vi "Data Publishing Service.vi"(10 "NIVS.Workspace Event":refnum<event-registration>, 11 "NIVS.Gateway IP Address":string="localhost") -> ()   [LabVIEW 2019, in "Data Publishing Service.lvlib"]
uses:
  Data Publishing Service.lvlib
  Types/State Variables.ctl
  Types/INI Configuration.ctl
  <vilib>/NI VeriStand/Execution/Workspace/WorkspaceAPI.ctl
  <vilib>/NI VeriStand/Execution/AlarmManager/AlarmManagerAPI.ctl
  <vilib>/Skyline/Tag/Wrapper/Wrapper_class/NI Skyline Tag.lvclass
  <vilib>/NI VeriStand/Execution/Alarm/AlarmAPI.ctl
  <vilib>/Platform/TimedLoop/XDataNode/timing_clust.ctl
  <vilib>/Platform/TimedLoop/XDataNode/nitl_modes.ctl
  <vilib>/Platform/TimedLoop/XDataNode/wakeup.ctl
  <vilib>/Skyline/Tag/Shared/typedefs/DataType.ctl
  <vilib>/Utility/error.llb/DialogType.ctl
  <vilib>/Skyline/Tag/Wrapper/Wrapper_class/Delete Tag (Multiple).vi
  <vilib>/platform/TimedLoop/XDataNode/XDataNode.xnode
  <vilib>/NI VeriStand/Execution/Workspace/NI_VS Workspace ExecutionAPI.lvlib
  <vilib>/Platform/TimedLoop/XDataNode/XDNodeRunTimeDep.lvlib
  <vilib>/Utility/SystemLogging/NI_SystemLogging.lvlib
  NationalInstruments.VeriStand.ClientAPI
  <vilib>/NI VeriStand/Execution/AlarmManager/NI_VS AlarmManager ExecutionAPI.lvlib
  <vilib>/NI VeriStand/Execution/Alarm/NI_VS Alarm ExecutionAPI.lvlib
  <vilib>/Skyline/Tag/Shared/NI Skyline Tag.lvlib
panel:
  out "Loop Rate":u32
  in  "Stop":bool
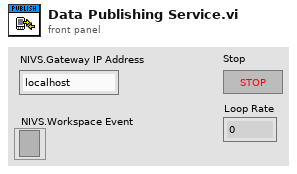
[diagram p1: front panel]
types:
  T1 = typedef "Data Publishing Service.lvlib/State Variables.ctl" = cluster{"INI":T2, "VS.Workspace.Ref":T3, "VS.AlarmManager.Ref":T4, "VS.Connected?":bool, "Tags.Deployed?":bool, "Tags.Initialized":bool, "Process.Name":string, "Aliases":string[], "Alias.Names":string[], "Alias.Tag.Paths":string[], "Alias.SysLink.Refs":refnum<class "NI Skyline Tag.lvclass">[], "Alarms":string[], "Alarm.Names":string[], "Alarm.Tag.Paths":string[], "Alarm.SysLink.Refs":refnum<class "NI Skyline Tag.lvclass">[], "Alarm.VS.Refs":T5[]}
  T2 = typedef "Data Publishing Service.lvlib/INI Configuration.ctl" = cluster{"Library.Name":string, "Alias.FolderPath":string, "Publish.Period_ms":u32, "Alias.Publish":bool, "Alarm.Publish":bool}
  T3 = typedef "NI_VS Workspace ExecutionAPI.lvlib/WorkspaceAPI.ctl" = refnum<k24>
  T4 = typedef "NI_VS AlarmManager ExecutionAPI.lvlib/AlarmManagerAPI.ctl" = refnum<k24>
  T5 = typedef "NI_VS Alarm ExecutionAPI.lvlib/AlarmAPI.ctl" = refnum<k24>
  T6 = typedef "NI_VS Workspace ExecutionAPI.lvlib/SystemStateEventRef.ctl" = cluster{"CustDatRef":refnum<user-event>, "EvtRef":refnum<k27>, "Target State User Event":refnum<user-event>}
  T7 = typedef "NI_VS Workspace ExecutionAPI.lvlib/SystemStateRegEventRef.ctl" = refnum<event-registration>
  T8 = cluster{"NIVS.Workspace Event":refnum<event-registration>, "SystemChangeEventRef":T7}
  T9 = typedef "XDNodeRunTimeDep.lvlib/timing_clust.ctl" = cluster{"Expected End [f-1]":u64, "Actual End [f-1]":u64, "Finished Late? [f-1]":bool, "Expected End [i-1]":u64, "Actual End [i-1]":u64, "Finished Late? [i-1]":bool, "Expected Start [i]":u64, "Actual Start [i]":u64, "Expected Start [f]":u64, "Actual Start [f]":u64, "Source Name":string, "Structure Name":string, "Period":i64, "Deadline":i64, "Offset":i64, "Start":i64, "Priority":i32, "Timeout":i32, "Mode":T10, "Wakeup Reason":T11, "Error":errorcluster, "Source Type":string, "Secondary Source Type":string, "Global End Time":u64, "Global Start Time":u64, "Frame Duration":u64, "Iteration Duration":u64, "Assigned CPU":i32, "I/O Scan Engine Mode":u32}
  T10 = typedef "XDNodeRunTimeDep.lvlib/nitl_modes.ctl" = enum32{"No Change", "Process missed periods, maintain original phase", "Discard missed periods, maintain original phase", "Process missed periods, ignore original phase", "Discard missed periods, ignore original phase"}
  T11 = typedef "XDNodeRunTimeDep.lvlib/wakeup.ctl" = enum32{"Normal", "Aborted", "Asynchronous wakeup", "Timing source error", "Timed loop error", "Timeout"}
  T12 = typedef "NI Skyline Tag.lvlib/DataType.ctl" = enum32{"Double", "I32", "String", "Boolean", "U64", "Timestamp"}
  T13 = typedef "NI_VS Workspace ExecutionAPI.lvlib/SystemState.ctl" = u8
  T14 = typedef "DialogType.ctl" = u16
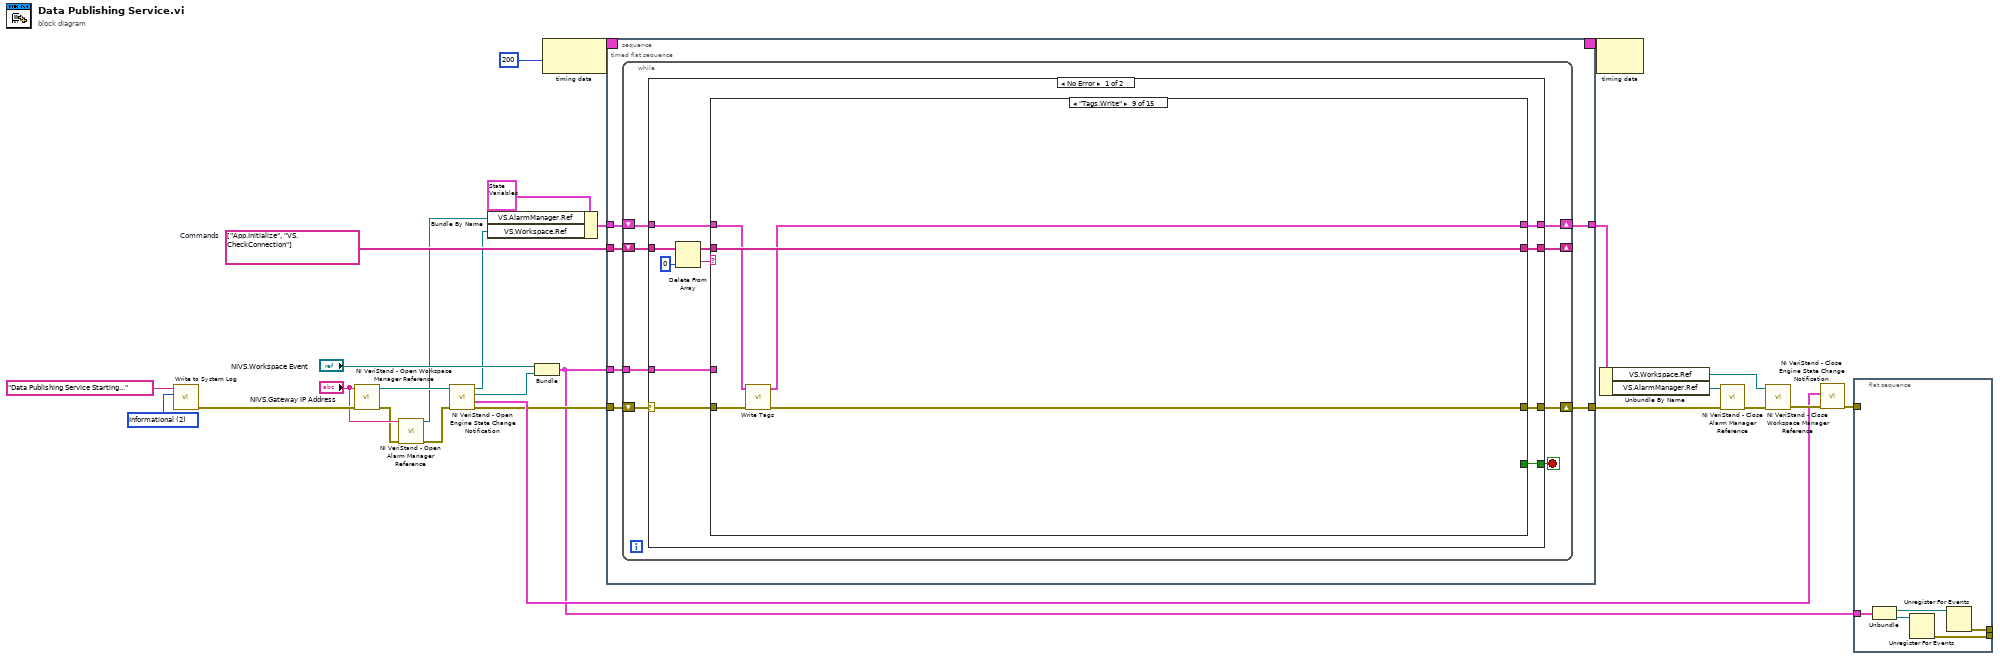
[diagram p0: block diagram]
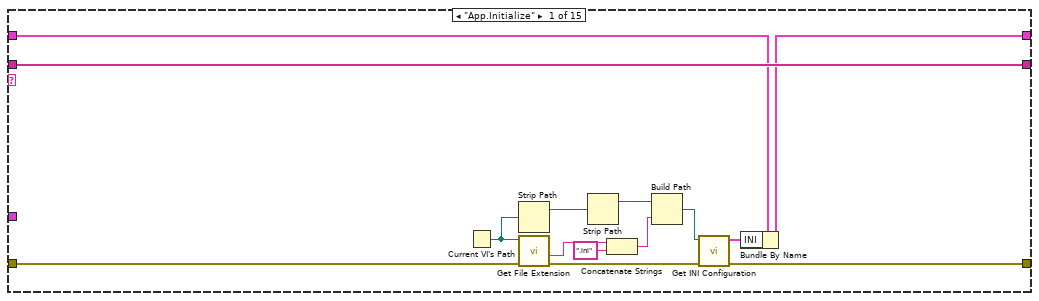
[diagram p2: hidden frame]
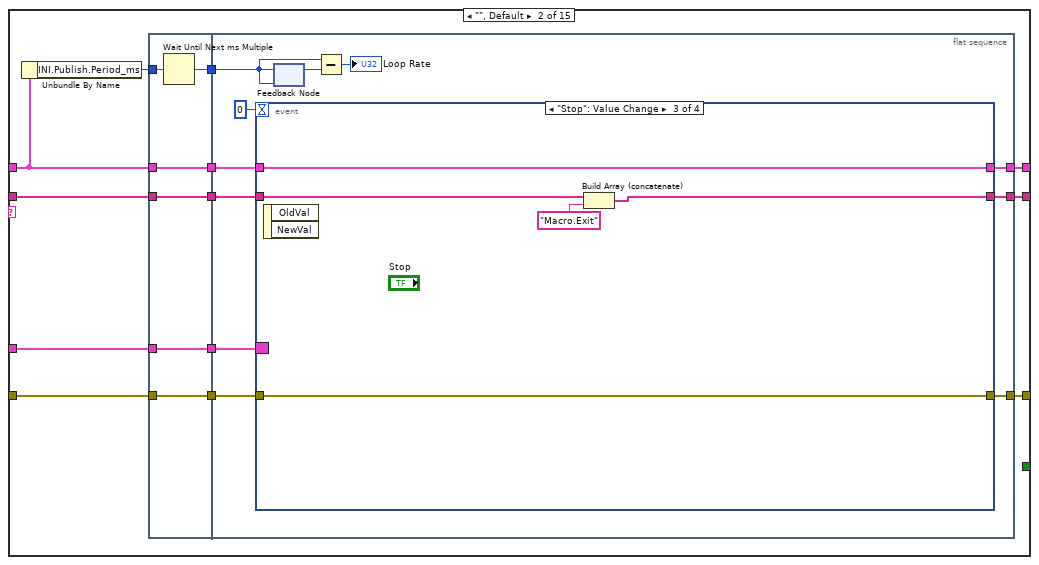
[diagram p3: hidden frame]
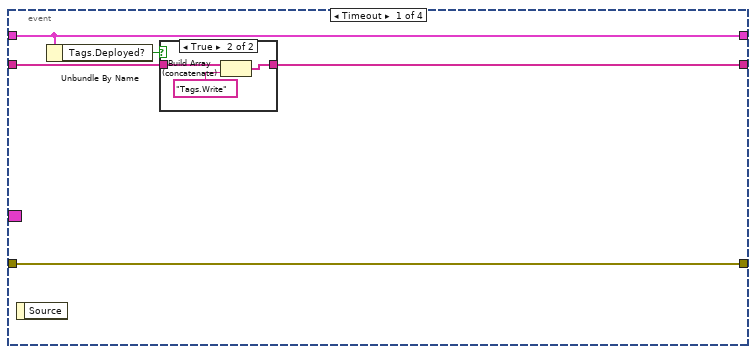
[diagram p4: hidden frame]
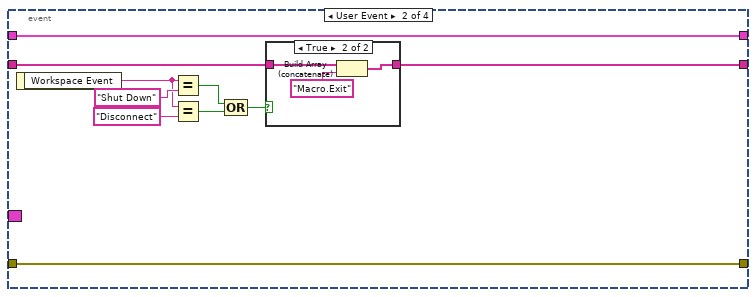
[diagram p6: hidden frame]
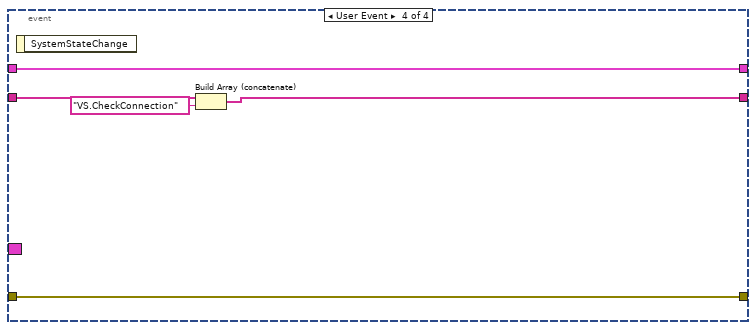
[diagram p8: hidden frame]
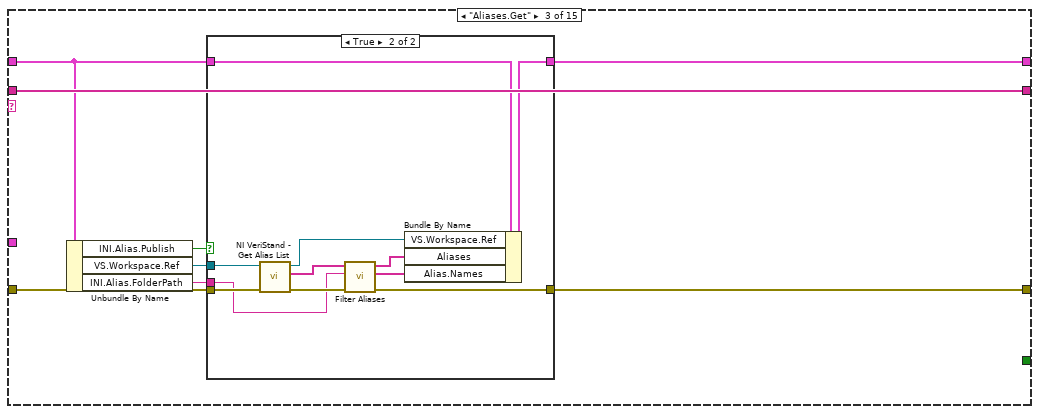
[diagram p9: hidden frame]
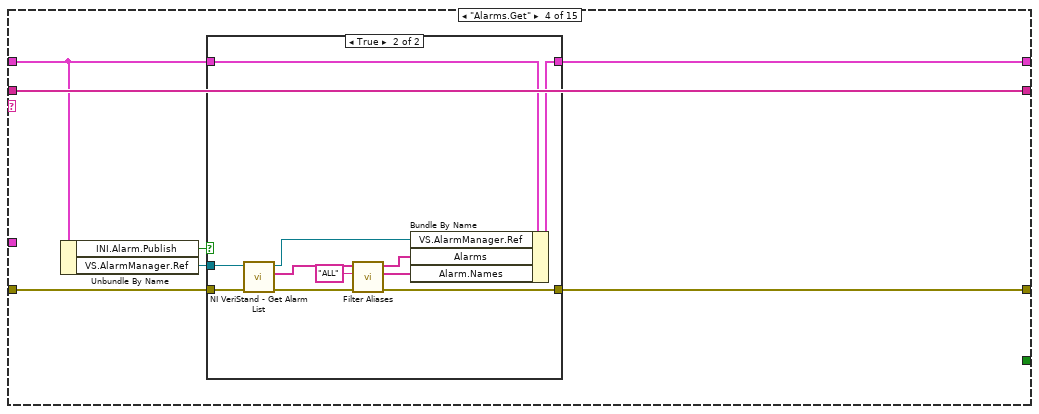
[diagram p11: hidden frame]
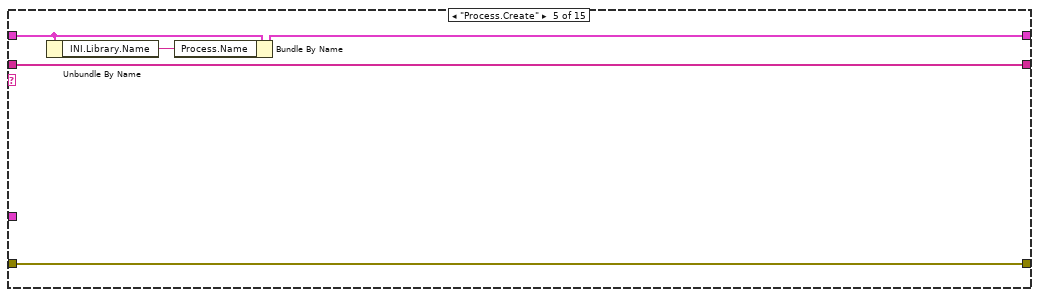
[diagram p13: hidden frame]
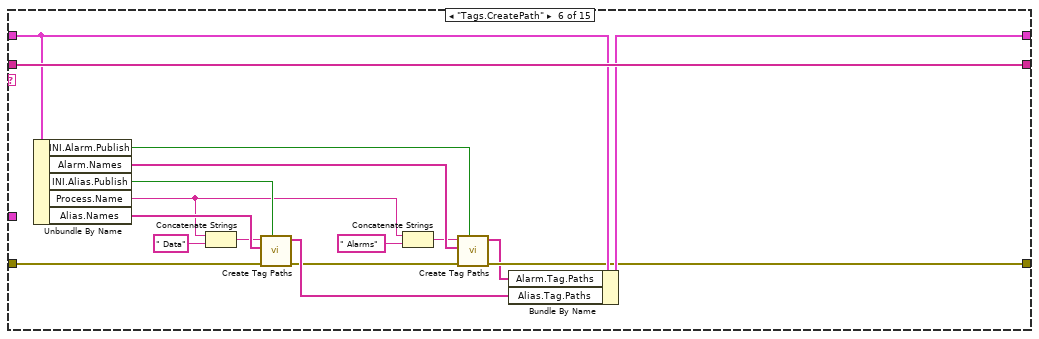
[diagram p14: hidden frame]
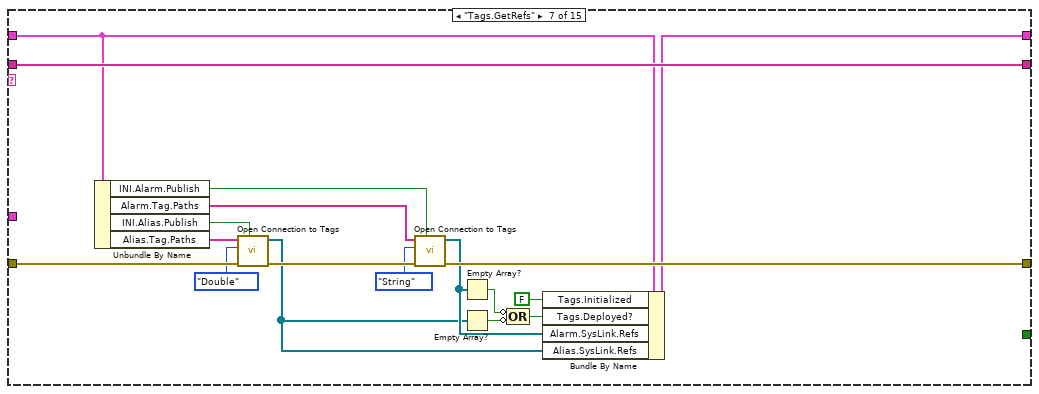
[diagram p15: hidden frame]
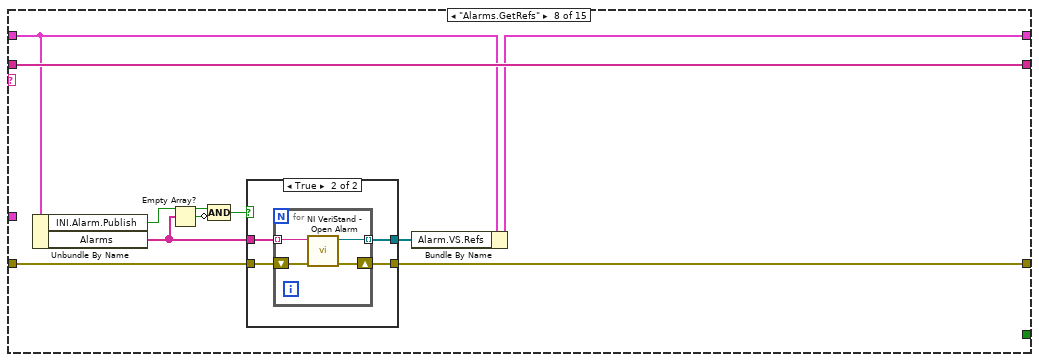
[diagram p16: hidden frame]
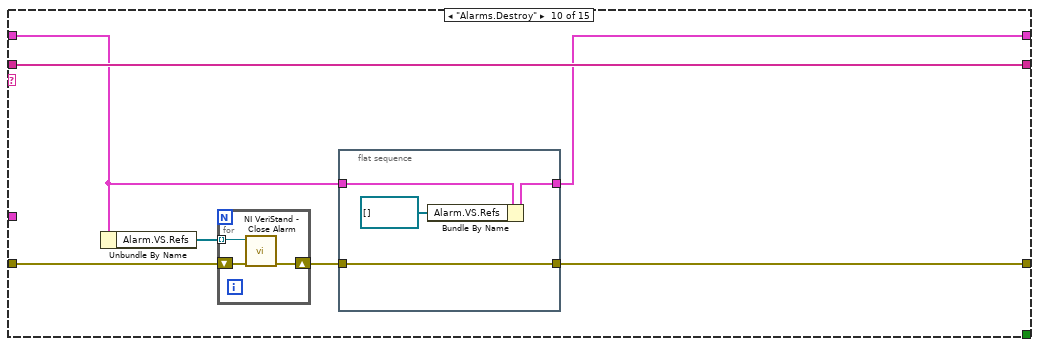
[diagram p18: hidden frame]
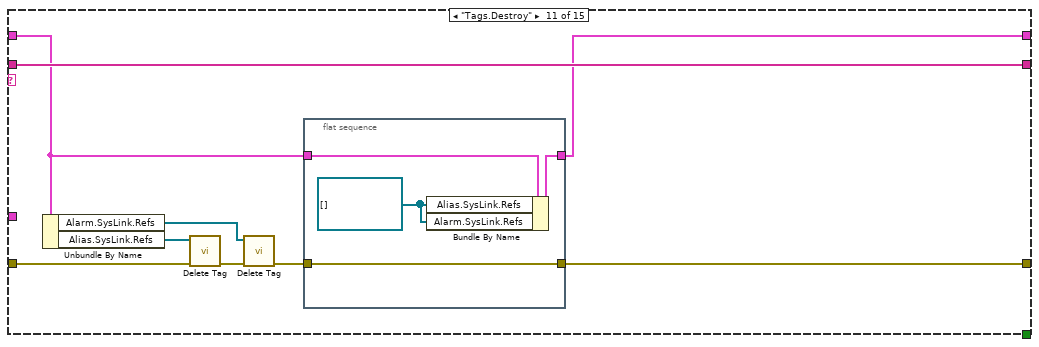
[diagram p19: hidden frame]
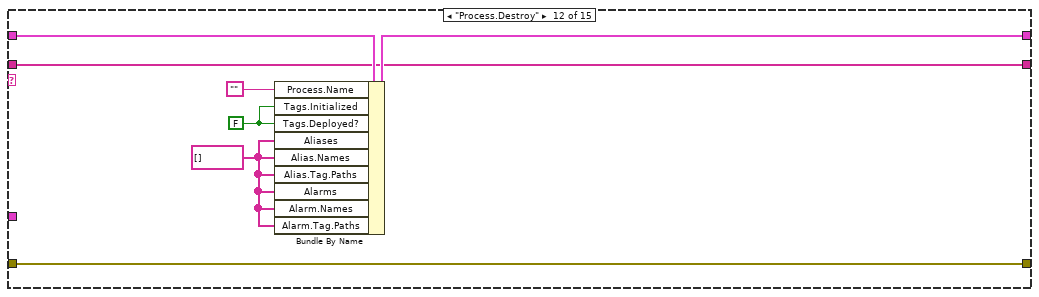
[diagram p20: hidden frame]
diagram:
  w9 = 2 items=["Error", "Warning", "Informational"] ("severity")
  w21 = string[] ["App.Initialize", "VS.CheckConnection"]  # Commands
  n1 = call <vilib>:"Write to System Log.vi"("severity"=w9, "message"="Data Publishing Service Starting...") -> ("error out"=w8:errorcluster)  [unwired: 9 in]
  n2 = call <vilib>:"NI VeriStand - Open Workspace Manager Reference.vi"("error in (no error)"=w8, "Gateway IP Address (\"\": localhost)"="NIVS.Gateway IP Address") -> ("error out"=w6:errorcluster, "WorkspaceManager"=w27:T3)  [unwired: 8 in]
  n3 = call <vilib>:"NI VeriStand - Open Alarm Manager Reference.vi"("error in (no error)"=w6, "Gateway IP Address (\"\": localhost)"="NIVS.Gateway IP Address") -> ("error out"=w5:errorcluster, "AlarmManager"=w4:T4)  [unwired: 8 in]
  n4 = call <vilib>:"NI VeriStand - Open Engine State Change Notification.vi"("error in (no error)"=w5, "WorkspaceManager in"=w27) -> ("error out"=w22:errorcluster, "SystemStateRefs"=w25:T6, "SystemChangeEventRef"=w23:T7, "WorkspaceManager out"=w18:T3)  [unwired: 6 in]
  n5 = Bundle By Name(cluster=T1 {"INI"={"Library.Name"="NI VeriStand Published Data", "Alias.FolderPath"="All", "Publish.Period_ms"=0, "Alias.Publish"=FALSE, "Alarm.Publish"=FALSE}, "VS.Workspace.Ref"=refnum, "VS.AlarmManager.Ref"=refnum, "VS.Connected?"=FALSE, "Tags.Deployed?"=FALSE, "Tags.Initialized"=FALSE, "Process.Name"="", "Aliases"=[], "Alias.Names"=[], "Alias.Tag.Paths"=[], "Alias.SysLink.Refs"=[], "Alarms"=[], "Alarm.Names"=[], "Alarm.Tag.Paths"=[], "Alarm.SysLink.Refs"=[], "Alarm.VS.Refs"=[]}, "VS.AlarmManager.Ref"=w4, "VS.Workspace.Ref"=w18) -> (w16:T1)
  n6 = Bundle("NIVS.Workspace Event"="NIVS.Workspace Event", "SystemChangeEventRef"=w23) -> (w20:T8)  [unwired: 1 in]
  n7 = node-c288(200 ("Priority")) -> (w13:T9)
  n8 = timed-sequence {
    timing: w13 -> [_]
    timing-out: [_] -> w12
    tunnel: [w33] -> w3
    tunnel: w22 -> [w32]
    tunnel: w21 -> [w31]
    tunnel: w20 -> [w30]
    tunnel: w16 -> [w29]
    tunnel: [w28] -> w15
    n9 = timed-flat-sequence {
      tunnel: [w39] -> w33
      tunnel: w32 -> [w38]
      tunnel: w31 -> [w37]
      tunnel: w30 -> [w36]
      tunnel: w29 -> [w35]
      tunnel: [w34] -> w28
      n10 = while {
        tunnel: w36 -> [w47]
        shift-right: [w46] -> w39
        shift-left: w38 -> [w44]
        shift-right: [w41] -> w34
        shift-left: w35 -> [w45]
        shift-right: [w42] -> _
        shift-left: w37 -> [w43]
        stop <- w40 stop-if-true
        n11 = case shown="No Error" w44 {
          selector: w44 -> [w54 w316]
          tunnel: w47 -> [w58 _]
          tunnel: [w57 w319] -> w46
          tunnel: [w56 _] -> w40
          tunnel: w45 -> [w55 w325]
          tunnel: w43 -> [w53 w324]
          tunnel: [w49 w324] -> w42
          tunnel: [w48 w325] -> w41
          frame No Error {
            n12 = Delete From Array(array=w53, index=0) -> (deleted portion=w51:string, array with subset deleted=w50:string[])  [unwired: 1 in]
            n13 = case shown="\"Tags.Write\"" w51 {
              tunnel: w58 -> [_ w85 _ _ _ _ _ _ _ _ _ _ _ _ _]
              tunnel: w54 -> [w59 w84 w141 w161 w181 w197 w215 w225 w239 w245 w262 w271 w289 w300 w309]
              tunnel: [w72 w83 w138 w158 w181 w191 w208 w224 w236 w242 w261 w271 w278 w300 w310] -> w57
              tunnel: [_ _ _ _ _ _ _ _ _ _ _ _ _ _ TRUE] -> w56
              tunnel: w55 -> [w70 w79 w140 w160 w178 w196 w207 w223 w237 w244 w259 w274 w287 w303 w313]
              tunnel: w50 -> [w71 w82 w142 w162 w179 w198 w216 w226 w240 w247 w263 w272 w282 w305 w312]
              tunnel: [w71 w81 w142 w162 w179 w198 w216 w226 w240 w247 w263 w272 w283 w304 w312] -> w49
              tunnel: [w68 w80 w143 w163 w180 w194 w206 w221 w238 w243 w258 w273 w286 w303 w313] -> w48
              frame "App.Initialize" {
                n14 = Current VI's Path() -> (path=w63:path)
                n15 = Strip Path(path=w63) -> (stripped path=w62:path)  [unwired: 1 out]
                n16 = call <vilib>:"Get File Extension.vi"("error in (no error)"=w59, "file"=w63) -> ("error out"=w67:errorcluster, "filename without extension"=w66:string)  [unwired: 5 in, 3 out]
                n17 = Strip Path(path=w62) -> (stripped path=w61:path)  [unwired: 1 out]
                n18 = Concatenate Strings(w66, ".ini" ("string")) -> (w64:string)
                n19 = Build Path(base path=w61, name or relative path=w64) -> (appended path=w60:path)
                n20 = call "Get INI Configuration.vi"("error in (no error)"=w67, "configuration file path"=w60) -> ("error out"=w72:errorcluster, "INI"=w69:T2)  [unwired: 8 in]
                n21 = Bundle By Name(cluster=w70, "INI"=w69) -> (w68:T1)
              }
              frame "", Default {
                n22 = Unbundle By Name(w79) -> ("INI.Publish.Period_ms"=w78:u32)
                n23 = flat-sequence {
                  tunnel: w78 -> [w87]
                  tunnel: w79 -> [w88]
                  tunnel: w82 -> [w89]
                  tunnel: w84 -> [w90]
                  tunnel: w85 -> [w91]
                  tunnel: [w91] -> w77
                  tunnel: [w90] -> w76
                  tunnel: [w89] -> w75
                  tunnel: [w88] -> w74
                  tunnel: [w86] -> w73
                  tunnel: [w100] -> w83
                  tunnel: [w98] -> w81
                  tunnel: [w97] -> w80
                  tunnel: w77 -> [w102]
                  tunnel: w76 -> [w101]
                  tunnel: w75 -> [w99]
                  tunnel: w74 -> [w96]
                  tunnel: w73 -> [w93]
                  frame #0 {
                    n24 = Wait Until Next ms Multiple(millisecond multiple=w87) -> (millisecond timer value=w86:u32)
                  }
                  frame #1 {
                    n25 = event shown="[2] \"Stop\": Value Change" {
                      selector: w102 -> [_ _ _ _]
                      dyn-events: _ -> [_ _ _ _]
                      timeout: 0 -> [_ _ _ _]
                      tunnel: w101 -> [w103 w121 w130 w135]
                      tunnel: [w103 w121 w130 w135] -> w100
                      tunnel: w96 -> [w104 w120 w129 w131]
                      tunnel: w99 -> [w105 w119 w128 w134]
                      tunnel: [w106 w117 w127 w133] -> w98
                      tunnel: [w104 w120 w129 w131] -> w97
                      event Timeout {
                        n26 = event-data() -> ()  [unwired: 1 in, 1 out]
                        n27 = Unbundle By Name(w104) -> ("Tags.Deployed?"=w107:bool)
                        n28 = case shown="True" w107 {
                          tunnel: w105 -> [w108 w110]
                          tunnel: [w108 w109] -> w106
                          frame False {
                          }
                          frame True {
                            n29 = Build Array (concatenate)(w110, "Tags.Write" ("y")) -> (w109:string[])
                          }
                        }
                      }
                      event User Event {
                        n30 = event-data() -> ("Workspace Event"=w112:string)  [unwired: 1 in]
                        n31 = Equal?(x=w112, y="Shut Down") -> (x = y?=w114:bool)
                        n32 = Equal?(x=w112, y="Disconnect") -> (x = y?=w115:bool)
                        n33 = Compound Arithmetic op=OR(w114, w115) -> (w113:bool)
                        n34 = case shown="True" w113 {
                          tunnel: w119 -> [w122 w125]
                          tunnel: [w122 w124] -> w117
                          frame False {
                          }
                          frame True {
                            n35 = Build Array (concatenate)(w125, "Macro.Exit" ("y")) -> (w124:string[])
                          }
                        }
                      }
                      event "Stop": Value Change {
                        n36 = event-data() -> ()  [unwired: 1 in, 2 out]
                        n37 = Build Array (concatenate)(w128, "Macro.Exit" ("y")) -> (w127:string[])
                      }
                      event User Event {
                        n38 = event-data() -> ()  [unwired: 1 in, 1 out]
                        n39 = Build Array (concatenate)(w134, "VS.CheckConnection") -> (w133:string[])
                      }
                    }
                    n40 = feedback-in #1(w93) -> ()
                    n41 = feedback #1(w93) -> (w94:u32)
                    n42 = Subtract(x=w93, y=w94) -> (x-y=→"Loop Rate":u32)
                  }
                }
              }
              frame "Aliases.Get" {
                n43 = Unbundle By Name(w140) -> ("INI.Alias.Publish"=w136:bool, "VS.Workspace.Ref"=w139:T3, "INI.Alias.FolderPath"=w137:string)
                n44 = case shown="True" w136 {
                  tunnel: [w144 w156] -> w143
                  tunnel: w141 -> [w145 w155]
                  tunnel: w140 -> [w144 w154]
                  tunnel: w139 -> [_ w153]
                  tunnel: [w145 w149] -> w138
                  tunnel: w137 -> [_ w147]
                  frame False {
                  }
                  frame True {
                    n45 = call <vilib>:"NI VeriStand - Get Alias List.vi"("error in (no error)"=w155, "WorkspaceManager in"=w153) -> ("error out"=w150:errorcluster, "Aliases"=w151:string[], "WorkspaceManager out"=w152:T3)  [unwired: 6 in, 1 out]
                    n46 = call "Filter Aliases.vi"("error in (no error)"=w150, "Folder Filter"=w147, "VS Paths in"=w151) -> ("error out"=w149:errorcluster, "Tag.Names"=w146:string[], "VS Paths out"=w148:string[])  [unwired: 6 in]
                    n47 = Bundle By Name(cluster=w154, "VS.Workspace.Ref"=w152, "Aliases"=w148, "Alias.Names"=w146) -> (w156:T1)
                  }
                }
              }
              frame "Alarms.Get" {
                n48 = Unbundle By Name(w160) -> ("INI.Alarm.Publish"=w157:bool, "VS.AlarmManager.Ref"=w159:T4)
                n49 = case shown="True" w157 {
                  tunnel: [w164 w176] -> w163
                  tunnel: w161 -> [w165 w170]
                  tunnel: w160 -> [w164 w175]
                  tunnel: w159 -> [_ w171]
                  tunnel: [w165 w174] -> w158
                  frame False {
                  }
                  frame True {
                    n50 = call <vilib>:"NI VeriStand - Get Alarm List.vi"("error in (no error)"=w170, "AlarmManager in"=w171) -> ("error out"=w169:errorcluster, "alarms"=w167:string[], "AlarmManager out"=w168:T4)  [unwired: 7 in]
                    n51 = call "Filter Aliases.vi"("error in (no error)"=w169, "Folder Filter"="ALL" ("Alias.FolderPath"), "VS Paths in"=w167) -> ("error out"=w174:errorcluster, "Tag.Names"=w172:string[], "VS Paths out"=w173:string[])  [unwired: 6 in]
                    n52 = Bundle By Name(cluster=w175, "VS.AlarmManager.Ref"=w168, "Alarms"=w173, "Alarm.Names"=w172) -> (w176:T1)
                  }
                }
              }
              frame "Process.Create" {
                n53 = Unbundle By Name(w178) -> ("INI.Library.Name"=w177:string)
                n54 = Bundle By Name(cluster=w178, "Process.Name"=w177) -> (w180:T1)
              }
              frame "Tags.CreatePath" {
                n55 = Unbundle By Name(w196) -> ("INI.Alarm.Publish"=w189:bool, "Alarm.Names"=w188:string[], "INI.Alias.Publish"=w193:bool, "Process.Name"=w183:string, "Alias.Names"=w187:string[])
                n56 = Concatenate Strings(w183, " Data" ("string")) -> (w186:string)
                n57 = call "Create Tag Paths.vi"("Create?"=w193, "error in (no error)"=w197, "Names in"=w187, "Process.Name"=w186) -> ("error out"=w192:errorcluster, "Names out"=w195:string[])  [unwired: 6 in]
                n58 = Concatenate Strings(w183, " Alarms" ("string")) -> (w182:string)
                n59 = call "Create Tag Paths.vi"("Create?"=w189, "error in (no error)"=w192, "Names in"=w188, "Process.Name"=w182) -> ("error out"=w191:errorcluster, "Names out"=w190:string[])  [unwired: 6 in]
                n60 = Bundle By Name(cluster=w196, "Alarm.Tag.Paths"=w190, "Alias.Tag.Paths"=w195) -> (w194:T1)
              }
              frame "Tags.GetRefs" {
                n61 = Unbundle By Name(w207) -> ("INI.Alarm.Publish"=w209:bool, "Alarm.Tag.Paths"=w210:string[], "INI.Alias.Publish"=w213:bool, "Alias.Tag.Paths"=w212:string[])
                n62 = call "Open Connection to Tags.vi"("Publish"=w213, "error in (no error)"=w215, "data type"=DataType."Double", "Tag.Paths"=w212) -> ("error out"=w211:errorcluster, "SysLink.Refs"=w204:refnum<class "NI Skyline Tag.lvclass">[])  [unwired: 6 in]
                n63 = call "Open Connection to Tags.vi"("Publish"=w209, "error in (no error)"=w211, "data type"=DataType."String", "Tag.Paths"=w210) -> ("error out"=w208:errorcluster, "SysLink.Refs"=w205:refnum<class "NI Skyline Tag.lvclass">[])  [unwired: 6 in]
                n64 = Empty Array?(array=w205) -> (empty?=w203:bool)
                n65 = Empty Array?(array=w204) -> (empty?=w202:bool)
                n66 = Compound Arithmetic op=OR(invert w203, invert w202) -> (w201:bool)
                n67 = Bundle By Name(cluster=w207, "Tags.Initialized"=FALSE, "Tags.Deployed?"=w201, "Alarm.SysLink.Refs"=w205, "Alias.SysLink.Refs"=w204) -> (w206:T1)
              }
              frame "Alarms.GetRefs" {
                n68 = Unbundle By Name(w223) -> ("INI.Alarm.Publish"=w217:bool, "Alarms"=w220:string[])
                n69 = Empty Array?(array=w220) -> (empty?=w219:bool)
                n70 = Compound Arithmetic op=AND(w217, invert w219) -> (w218:bool)
                n71 = case shown="True" w218 {
                  tunnel: w225 -> [w227 w231]
                  tunnel: w220 -> [_ w230]
                  tunnel: [w227 w229] -> w224
                  tunnel: [_ w228] -> w222
                  frame False {
                  }
                  frame True {
                    n72 = for {
                      tunnel: w230 -> [w234] mode=indexing
                      tunnel: [w233] -> w228 mode=indexing
                      shift-right: [w232] -> w229
                      shift-left: w231 -> [w235]
                      n73 = call <vilib>:"NI VeriStand - Open Alarm.vi"("error in (no error)"=w235, "Alarm Name"=w234) -> ("error out"=w232:errorcluster, "Alarm"=w233:T5)  [unwired: 8 in]
                    }
                  }
                }
                n74 = Bundle By Name(cluster=w223, "Alarm.VS.Refs"=w222) -> (w221:T1)
              }
              frame "Tags.Write" {
                n75 = call "Write Tags.vi"("error in (no error)"=w239, "Cluster in"=w237) -> ("error out"=w236:errorcluster, "Cluster out"=w238:T1)  [unwired: 8 in]
              }
              frame "Alarms.Destroy" {
                n76 = Unbundle By Name(w244) -> ("Alarm.VS.Refs"=w246:T5[])
                n77 = for {
                  tunnel: w246 -> [w254] mode=indexing
                  shift-right: [w252] -> w241
                  shift-left: w245 -> [w253]
                  n78 = call <vilib>:"NI VeriStand - Close Alarm.vi"("error in (no error)"=w253, "Alarm"=w254) -> ("error out"=w252:errorcluster)  [unwired: 9 in]
                }
                n79 = flat-sequence {
                  tunnel: w244 -> [w251]
                  tunnel: [w250] -> w243
                  tunnel: [w249] -> w242
                  tunnel: w241 -> [w249]
                  frame #0 {
                    n80 = Bundle By Name(cluster=w251, "Alarm.VS.Refs"=T5[] []) -> (w250:T1)
                  }
                }
              }
              frame "Tags.Destroy" {
                n81 = Unbundle By Name(w259) -> ("Alarm.SysLink.Refs"=w255:refnum<class "NI Skyline Tag.lvclass">[], "Alias.SysLink.Refs"=w260:refnum<class "NI Skyline Tag.lvclass">[])
                n82 = call-poly <vilib>:"Delete Tag.vi"("error in (no error)"=w262, "tags"=w260) -> ("error out"=w257:errorcluster)  [unwired: 9 in]
                n83 = call-poly <vilib>:"Delete Tag.vi"("error in (no error)"=w257, "tags"=w255) -> ("error out"=w256:errorcluster)  [unwired: 9 in]
                n84 = flat-sequence {
                  tunnel: w259 -> [w267]
                  tunnel: [w266] -> w258
                  tunnel: [w265] -> w261
                  tunnel: w256 -> [w265]
                  frame #0 {
                    w264 = refnum<class "NI Skyline Tag.lvclass">[] [] ("SkyLine.Refs")
                    n85 = Bundle By Name(cluster=w267, "Alias.SysLink.Refs"=w264, "Alarm.SysLink.Refs"=w264) -> (w266:T1)
                  }
                }
              }
              frame "Process.Destroy" {
                w268 = string[] [] ("Aliases")
                w269 = FALSE ("SV.Deployed?")
                n86 = Bundle By Name(cluster=w274, "Process.Name"="", "Tags.Initialized"=w269, "Tags.Deployed?"=w269, "Aliases"=w268, "Alias.Names"=w268, "Alias.Tag.Paths"=w268, "Alarms"=w268, "Alarm.Names"=w268, "Alarm.Tag.Paths"=w268) -> (w273:T1)
              }
              frame "VS.CheckConnection" {
                w280 = 2 items=["Error", "Warning", "Informational"] ("severity")
                n87 = Unbundle By Name(w287) -> ("Tags.Deployed?"=w281:bool, "VS.Workspace.Ref"=w288:T3)
                n88 = call <vilib>:"NI VeriStand - Get System State.vi"("error in (no error)"=w289, "WorkspaceManager in"=w288) -> ("error out"=w279:errorcluster, "System State"=w285:T13)  [unwired: 5 in, 3 out]
                n89 = Greater Than 0?(x=w285) -> (x > 0?=w284:bool)
                n90 = case shown="True" w284 {
                  tunnel: [w292 w298] -> w283
                  tunnel: w282 -> [w293 w299]
                  tunnel: w281 -> [w291 _]
                  tunnel: ["- VeriStand Disconnected..." "- VeriStand Connected..."] -> w276
                  frame False {
                    n91 = case shown="True" w291 {
                      tunnel: [_ string[] ["Alarms.Destroy", "Tags.Destroy", "Process.Destroy"]] -> w294
                      frame False {
                      }
                      frame True {
                      }
                    }
                    n92 = Build Array (concatenate)(w293, w294) -> (w292:string[])
                  }
                  frame True {
                    n93 = Build Array (concatenate)(w299, string[] ["App.Initialize", "Aliases.Get", "Alarms.Get", "Process.Create", "Tags.CreatePath", "Tags.GetRefs", "Alarms.GetRefs"]) -> (w298:string[])
                  }
                }
                n94 = Bundle By Name(cluster=w287, "VS.Connected?"=w284) -> (w286:T1)
                n95 = Concatenate Strings("Data Publishing Service " ("message"), w276) -> (w275:string)
                n96 = call <vilib>:"Write to System Log.vi"("error in (no error)"=w279, "severity"=w280, "message"=w275) -> ("error out"=w278:errorcluster)  [unwired: 8 in]
              }
              frame "Macro.Exit" {
                n97 = Unbundle By Name(w303) -> ("Tags.Deployed?"=w301:bool)
                n98 = case shown="True" w301 {
                  tunnel: [string[] ["Exit"] string[] ["Alarms.Destroy", "Tags.Destroy", "Process.Destroy", "Exit"]] -> w302
                  frame False {
                  }
                  frame True {
                  }
                }
                n99 = Build Array (concatenate)(w305, w302) -> (w304:string[])
              }
              frame "Exit" {
                w311 = 2 items=["Error", "Warning", "Informational"] ("severity")
                n100 = call <vilib>:"Write to System Log.vi"("error in (no error)"=w309, "severity"=w311, "message"="Data Publishing Service Exiting...") -> ("error out"=w310:errorcluster)  [unwired: 8 in]
              }
            }
          }
          frame Error {
            w321 = T14 1 items=["no dialog", "OK message", "continue or stop message", "OK message + warnings", "continue/stop + warnings"] ("type of dialog (OK msg:1)")
            n101 = call <vilib>:"Clear Errors.vi"("error in (no error)"=w316, "specific error code to clear (0: all)"=-307650) -> ("error out"=w315:errorcluster)  [unwired: 4 in, 1 out]
            n102 = call <vilib>:"Clear Errors.vi"("error in (no error)"=w315, "specific error code to clear (0: all)"=-307654) -> ("error out"=w323:errorcluster)  [unwired: 4 in, 1 out]
            n103 = call <vilib>:"Simple Error Handler.vi"("type of dialog (OK msg:1)"=w321, "error in (no error)"=w323) -> ("error out"=w318:errorcluster, "message"=w320:string)  [unwired: 3 in, 3 out]
            n104 = case shown="Error .." w318 {
              selector: w318 -> [w326 _]
              tunnel: w320 -> [_ w329]
              tunnel: [w326 w327] -> w319
              frame No Error {
              }
              frame Error {
                w330 = 0 items=["Error", "Warning", "Informational"] ("severity")
                n105 = call <vilib>:"Write to System Log.vi"("severity"=w330, "message"=w329) -> ("error out"=w328:errorcluster)  [unwired: 9 in]
                n106 = call <vilib>:"Clear Errors.vi"("error in (no error)"=w328) -> ("error out"=w327:errorcluster)  [unwired: 5 in, 1 out]
              }
            }
          }
        }
      }
    }
  }
  n107 = node-c288(w12) -> ()  [unwired: 1 out]
  n108 = Unbundle By Name(w15) -> ("VS.Workspace.Ref"=w14:T3, "VS.AlarmManager.Ref"=w1:T4)
  n109 = call <vilib>:"NI VeriStand - Close Alarm Manager Reference.vi"("error in (no error)"=w3, "AlarmManager"=w1) -> ("error out"=w2:errorcluster)  [unwired: 9 in]
  n110 = call <vilib>:"NI VeriStand - Close Workspace Manager Reference.vi"("error in (no error)"=w2, "WorkspaceManager"=w14) -> ("error out"=w26:errorcluster)  [unwired: 9 in]
  n111 = call <vilib>:"NI VeriStand - Close Engine State Change Notification.vi"("error in (no error)"=w26, "SystemStateRefs"=w25) -> ("error out"=w19:errorcluster)  [unwired: 9 in]
  n112 = flat-sequence {
    tunnel: w20 -> [w335]
    tunnel: w19 -> [_]
    tunnel: [w334] -> _
    tunnel: [w333] -> _
    frame #0 {
      n113 = Unbundle(w335) -> ("NIVS.Workspace Event"=w336:refnum<event-registration>, "SystemChangeEventRef"=w337:T7)
      n114 = Unregister For Events(event registration refnum=w337) -> (error out=w333:errorcluster)  [unwired: 1 in]
      n115 = Unregister For Events(event registration refnum=w336) -> (error out=w334:errorcluster)  [unwired: 1 in]
    }
  }
